vi "高速脉冲绘制.vi"(8 "曲线设置":T2, 10 "历史数据":T3[](array[typedef]), 11 "映射方式":T1) -> (0 "曲线属性":cluster{"曲线名":string, "曲线颜色":u32, "线条宽度":u8}[](array[cluster]), 3 "XY图":cluster{"数据":dbl[], "数据":dbl[]}[](array[cluster]))   [LabVIEW 2020, in "数据显示.xctl"]
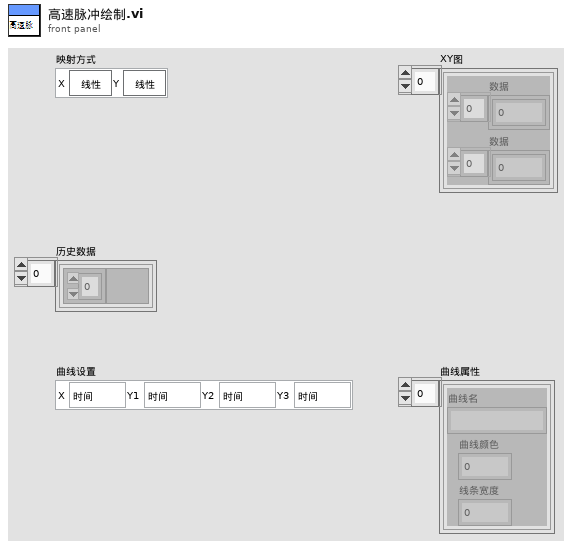
[diagram p1: front panel]
types:
  T1 = typedef "数据显示.xctl/映射方式.ctl" = cluster{"X":bool, "Y":bool}
  T2 = typedef "数据显示.xctl/曲线设置.ctl" = cluster{"X":enum16{"时间", "设置电压", "读取电流", "读取电压"}, "Y1":enum16{"时间", "设置电压", "读取电流", "读取电压"}, "Y2":enum16{"时间", "设置电压", "读取电流", "读取电压", "无"}, "Y3":enum16{"时间", "设置电压", "读取电流", "读取电压", "无"}}
  T3 = typedef "数据显示.xctl/波形数据定义.ctl" = cluster{"波形":dbl[][], "属性":variant}
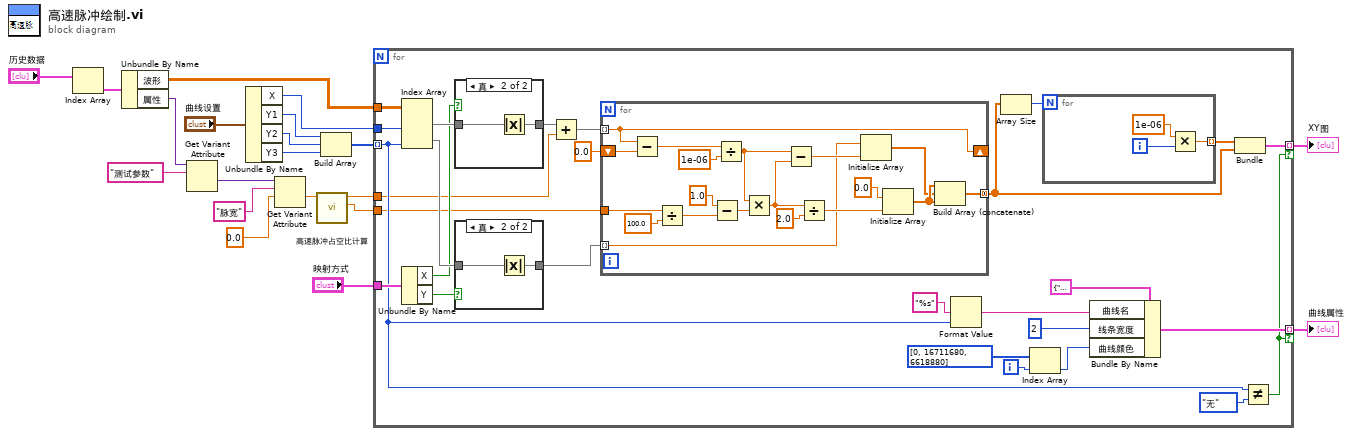
[diagram p0: block diagram]
diagram:
  n1 = Index Array(array="历史数据") -> (element=w17:T3)  [unwired: 1 in]
  n2 = Unbundle By Name(w17) -> ("波形"=w18:dbl[][], "属性"=w2:variant)
  n3 = Get Variant Attribute(Variant=w2, name="测试参数" ("名称")) -> (value=w3:variant)  [unwired: 2 in, 3 out]
  n4 = Unbundle By Name("曲线设置") -> ("X"=w11:enum16{"时间", "设置电压", "读取电流", "读取电压"}, "Y1"=w12:enum16{"时间", "设置电压", "读取电流", "读取电压"}, "Y2"=w13:enum16{"时间", "设置电压", "读取电流", "读取电压", "无"}, "Y3"=w14:enum16{"时间", "设置电压", "读取电流", "读取电压", "无"})
  n5 = Get Variant Attribute(Variant=w3, name="脉宽" ("名称"), default value (empty Variant)=0.0) -> (value=w6:dbl)  [unwired: 1 in, 3 out]
  n6 = call "高速脉冲占空比计算.vi"("脉宽"=w6) -> ("占空比"=w5:dbl, "周期"=w4:dbl)  [unwired: 9 in]
  n7 = Build Array(w12, w13, w14) -> (w15:enum16{"时间", "设置电压", "读取电流", "读取电压", "无"}[])
  n8 = for {
    tunnel: w18 -> [w48]
    tunnel: w11 -> [w25]
    tunnel: w15 -> [w24] mode=indexing
    tunnel: "映射方式" -> [w47]
    tunnel: [w41] -> w20 mode=indexing if=w37
    tunnel: [w40] -> w19 mode=indexing if=w37
    tunnel: w5 -> [w23]
    tunnel: w4 -> [w21]
    i -> [w35]
    n9 = Index Array(array=w48, index (col) #1=w25, index (col) #2=w24) -> (element #1=w46:dbl[], element #2=w45:dbl[])  [unwired: 2 in]
    n10 = Unbundle By Name(w47) -> ("X"=w44:bool, "Y"=w43:bool)
    n11 = case shown="真" w44 {
      tunnel: w46 -> [w74 w76]
      tunnel: [w74 w75] -> w27
      frame False {
      }
      frame True {
        n12 = Absolute Value(x=w76) -> (abs(x)=w75:dbl[])
      }
    }
    n13 = case shown="真" w43 {
      tunnel: w45 -> [w71 w73]
      tunnel: [w71 w72] -> w26
      frame False {
      }
      frame True {
        n14 = Absolute Value(x=w73) -> (abs(x)=w72:dbl[])
      }
    }
    n15 = Add(x=w27, y=w21) -> (x+y=w22:dbl[])
    n16 = for {
      tunnel: [w52] -> w30 mode=concatenating
      shift-right: [w67] -> _
      shift-left: 0.0 -> [w69]
      tunnel: w22 -> [w67] mode=indexing
      tunnel: w26 -> [w53] mode=indexing
      tunnel: w23 -> [w56]
      n17 = Subtract(x=w67, y=w69) -> (x-y=w68:dbl)
      n18 = Divide(x=w56, y=100.0) -> (x/y=w60:dbl)
      n19 = Subtract(x=1.0, y=w60) -> (x-y=w61:dbl)
      n20 = Divide(x=w68, y=1e-06) -> (x/y=w55:dbl)
      n21 = Multiply(x=w55, y=w61) -> (x*y=w64:dbl)
      n22 = Subtract(x=w55, y=w64) -> (x-y=w62:dbl)
      n23 = Divide(x=w64, y=2.0) -> (x/y=w65:dbl)
      n24 = Initialize Array(w53, w62) -> (w63:dbl[])
      n25 = Initialize Array(0.0, w65) -> (w66:dbl[])
      n26 = Build Array (concatenate)(w66, w63, w66) -> (w52:dbl[])
    }
    n27 = Format Value(format string="%s" ("格式字符串"), value (0)=w24) -> (output string=w32:string)  [unwired: 1 in]
    n28 = Array Size(array=w30) -> (size(s)=w31:i32)
    n29 = Index Array(array=u32[] [0, 16711680, 6618880], index=w35) -> (element=w34:u32)
    n30 = for {
      N: w31 -> [_]
      tunnel: [w49] -> w28 mode=indexing
      i -> [w50]
      n31 = Multiply(x=1e-06 ("y"), y=w50) -> (x*y=w49:dbl)
    }
    n32 = Bundle By Name(cluster=cluster{"曲线名":string, "曲线颜色":u32, "线条宽度":u8} {"曲线名"="", "曲线颜色"=0, "线条宽度"=0} ("曲线属性"), "曲线名"=w32, "线条宽度"=u8 2, "曲线颜色"=w34) -> (w40:cluster{"曲线名":string, "曲线颜色":u32, "线条宽度":u8})
    n33 = Bundle(w28, w30) -> (w41:cluster{dbl[], dbl[]})  [unwired: 1 in]
    n34 = Not Equal?(x=w24, y=enum16{"时间", "设置电压", "读取电流", "读取电压", "无"}."无") -> (x != y?=w37:bool)
  }
  "XY图" <- w20
  "曲线属性" <- w19
